vi "Get AVA Info wrapper.vi"(6 "pDummyAvaInfoOut":T1, 7 "bAckEna":i32, 8 "error in (no error)":errorcluster caption="错误输入（无错误）", 9 "pDummyAvaInfoIn":T1, 10 "dwCanNodeId":u32, 11 "dwDevIndex":u32) -> (0 "error out":errorcluster caption="错误输出", 1 "pDummyAvaInfoIn out":T1, 3 "function return":u32, 4 "pDummyAvaInfoOut out":T1)   [LabVIEW 2016, in "UISimCanFunc_wrapper.lvlib"]
doc: "_declspec (dllexport) DWORD GetAVAInfo_wrapper(DWORD dwDevIndex, DWORD dwCanNodeId,\n P_DUMMY_AVA_INFO_OBJ pDummyAvaInfoIn, BOOL bAckEna, P_DUMMY_AVA_INFO_OBJ pDummyAvaInfoOut);"
uses:
  <userlib>/UISimCanFunc_wrapper/UISimCanFunc_wrapper.lvlib
  <userlib>/UISimCanFunc_wrapper/UISimCanFunc_wrapper.dll
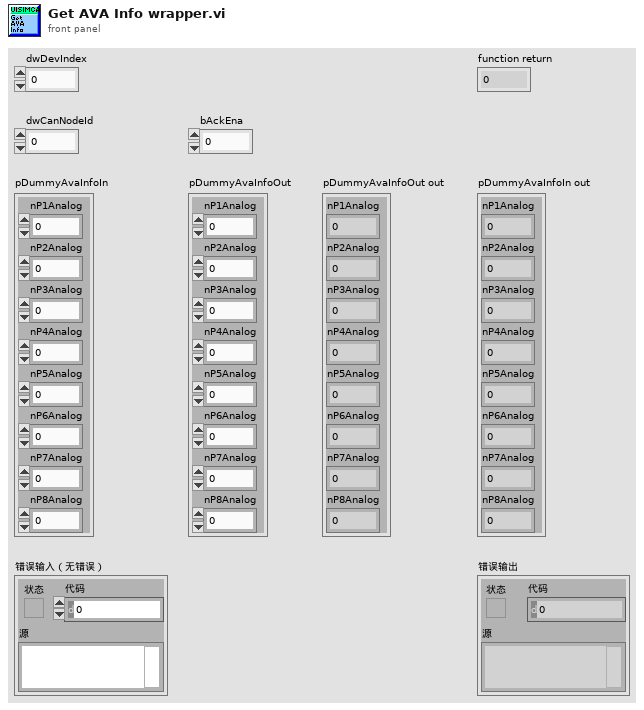
[diagram p1: front panel]
types:
  T1 = cluster{"nP1Analog":i32, "nP2Analog":i32, "nP3Analog":i32, "nP4Analog":i32, "nP5Analog":i32, "nP6Analog":i32, "nP7Analog":i32, "nP8Analog":i32}
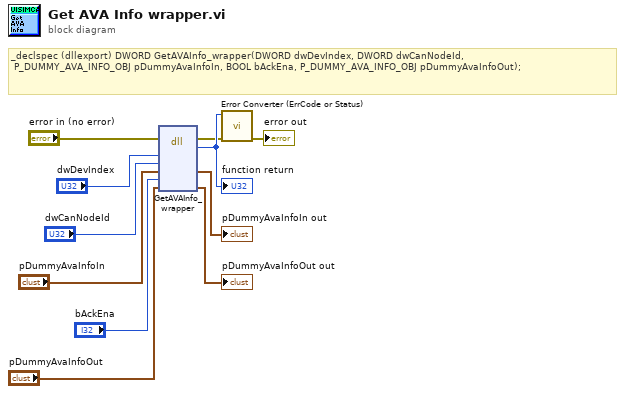
[diagram p0: block diagram]
diagram:
  # "_declspec (dllexport) DWORD GetAVAInfo_wrapper(DWORD dwDevIndex, DWORD dwCanNodeId,\n\tP_DUMMY_AVA_INFO_OBJ pDummyAvaInfoIn, BOOL bAckEna, P_DUMMY_AVA_INFO_OBJ pDummyAvaInfoOut);"
  n1 = dll-call lib="C:/Program Files (x86)/National Instruments/LabVIEW 2016/user.lib/UISimCanFunc_wrapper/UISimCanFunc_wrapper.*" fn="GetAVAInfo_wrapper"(error in="error in (no error)", "dwDevIndex"="dwDevIndex", "dwCanNodeId"="dwCanNodeId", "pDummyAvaInfoIn"="pDummyAvaInfoIn", "bAckEna"="bAckEna", "pDummyAvaInfoOut"="pDummyAvaInfoOut") -> (error out=w2:errorcluster, w11:u32, "pDummyAvaInfoIn"=→"pDummyAvaInfoIn out":T1, "pDummyAvaInfoOut"=→"pDummyAvaInfoOut out":T1)  [unwired: 5 in, 1 out]
  "function return" <- w11
  n2 = call <userlib>:"Error Converter (ErrCode or Status).vi"("error in (no error)"=w2, "error code"=w11) -> ("error out"=→"error out":errorcluster)  [unwired: 9 in]
